vi "configure.vi"(8 "error in (no error)":errorcluster, 11 "DL090202FPGAClock in":refnum<class "ClockDL090202FPGA.lvclass">) -> (0 "error out":errorcluster, 3 "DL090202FPGAClock out":refnum<class "ClockDL090202FPGA.lvclass">)   [LabVIEW 2010, in "ClockDL090202FPGA.lvclass"]
uses:
  ClockDL090202FPGA.lvclass
  type_enum.ctl
  common/xcontrols/XComponentSpecification/XComponentSpecification/XComponentSpecification.xctl
  ClockDL090202FPGA.lvclass/ClockDL090202FPGA.ctl
  FPGAWrapper/GenericFPGAWrapper/GenericFPGAWrapper/GenericFPGAWrapper.lvclass
  common/classes/ErrorController/ErrorController/class_data.vi
  common/classes/GenericComponent/GenericComponent/GenericComponent.lvclass
  common/classes/ErrorController/ErrorController/ErrorController.lvclass
panel:
  in  "FPGAWrapper spec":T1(xcontrol)
  out "Configuration name":string
  in  "type":T2
  in  "cancel":bool
  in  "save":bool
  # "Configure ClockDL090202FPGA"
  # "FPGAWrapper"
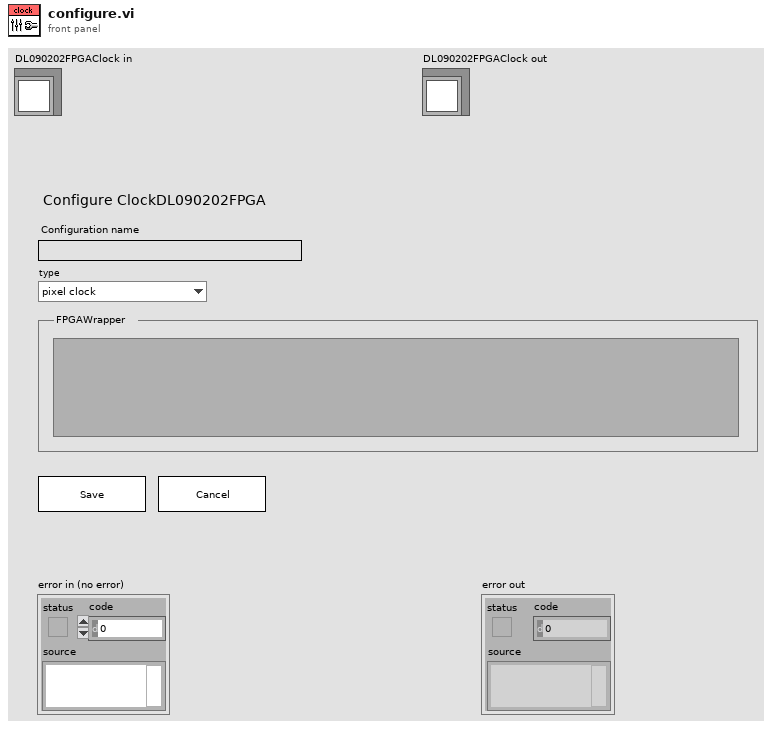
[diagram p1: front panel]
types:
  T1 = cluster{"class path":string, "configuration":string, "label":string, "settings name":string}
  T2 = typedef "ClockDL090202FPGA.lvclass/type_enum.ctl" = enum16{"pixel clock", "gate 1", "gate 2", "gate 3"}
  T3 = typedef "plugin_specification.ctl" = cluster{"class path":string, "configuration":string, "label":string, "settings name":string}
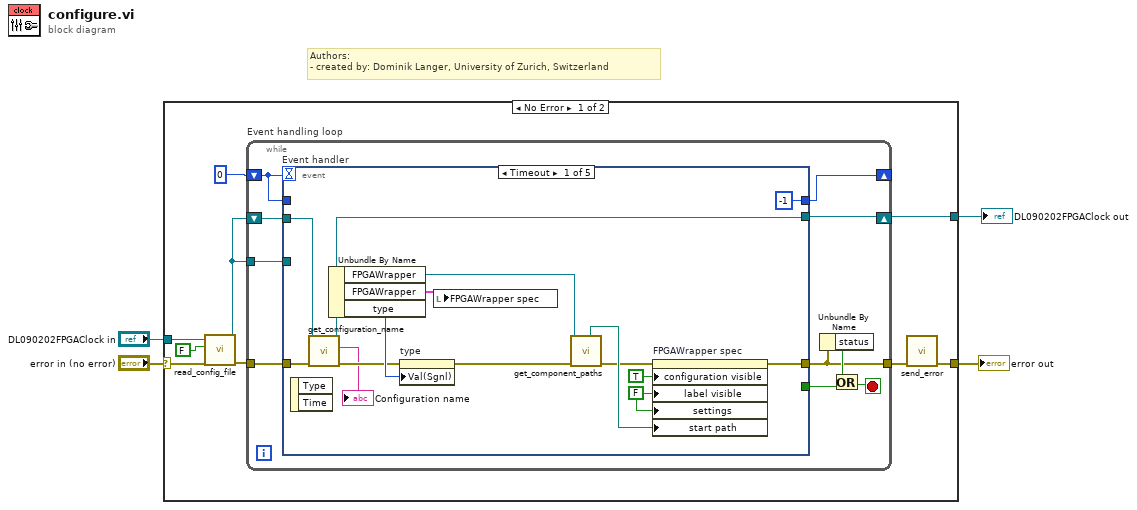
[diagram p0: block diagram]
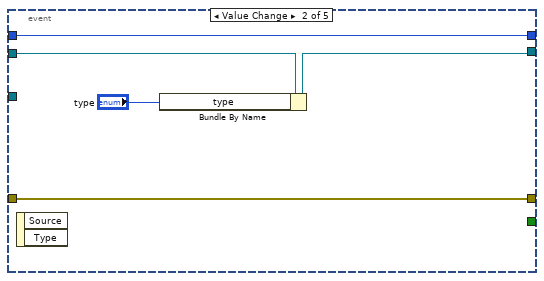
[diagram p2: hidden frame]
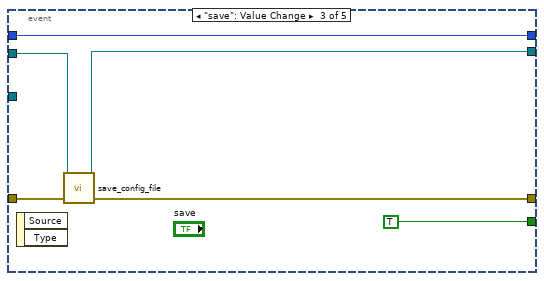
[diagram p3: hidden frame]
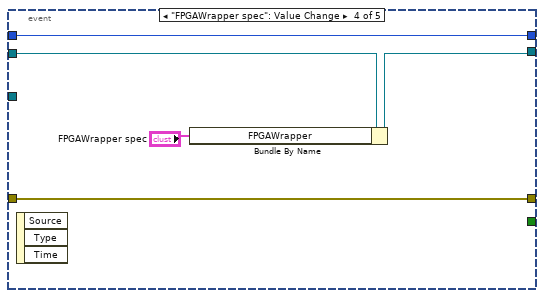
[diagram p4: hidden frame]
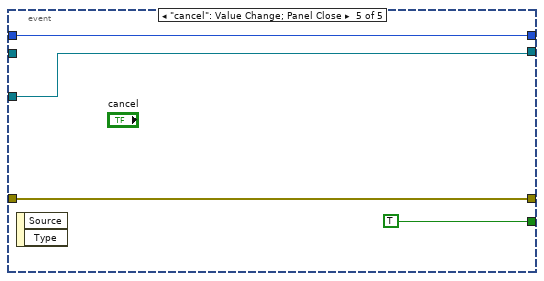
[diagram p5: hidden frame]
diagram:
  # "Authors: \n- created by: Dominik Langer, University of Zurich, Switzerland"
  n1 = case shown="No Error" "error in (no error)" {
    selector: "error in (no error)" -> [w11 w60]
    tunnel: [w7 w60] -> w3
    tunnel: [w12 w59] -> w1
    tunnel: "DL090202FPGAClock in" -> [w9 w59]
    frame No Error {
      n2 = call-dynamic "read_config_file.vi"("error in (no error)"=w11, "force load?"=FALSE, "GenericPlugin in"=w9) -> ("error out"=w10:errorcluster, "GenericPlugin out"=w5:refnum<class "ClockDL090202FPGA.lvclass">)  [unwired: 7 out]
      n3 = while "Event handling loop" {
        shift-right: [w21] -> _
        shift-left: 0 -> [w22]
        shift-right: [w19] -> w12
        shift-left: w5 -> [w20]
        tunnel: w10 -> [w23]
        tunnel: [w15] -> w6
        tunnel: w5 -> [w14]
        stop <- w17 stop-if-true
        n4 = event "Event handler" shown="[0] Timeout" {
          selector: _ -> [_ _ _ _ _]
          dyn-events: _ -> [_ _ _ _ _]
          timeout: w22 -> [_ _ _ _ _]
          tunnel: w23 -> [w36 w39 w48 w53 w57]
          tunnel: [-1 w43 w49 w54 w58] -> w21
          tunnel: w22 -> [_ w43 w49 w54 w58]
          tunnel: [w31 w39 w47 w53 w57] -> w15
          tunnel: [_ _ TRUE _ TRUE] -> w16
          tunnel: w20 -> [w34 w42 w44 w52 _]
          tunnel: [w25 w41 w46 w51 w55] -> w19
          tunnel: w14 -> [_ _ _ _ w55]
          event Timeout {
            w29 = FALSE ("label visible")
            n5 = event-data() -> ()  [unwired: 3 out]
            n6 = call "get_configuration_name.vi"("error in (no error)"=w36, "GenericPlugin.lvclass in"=w34) -> ("error out"=w35:errorcluster, "configuration name"=→"Configuration name":string, "GenericPlugin.lvclass out"=w25:refnum<class "ClockDL090202FPGA.lvclass">)  [unwired: 7 in]
            n7 = Unbundle By Name(w25) -> ("FPGAWrapper"=w24:refnum<class "GenericFPGAWrapper.lvclass">, "FPGAWrapper"=w32:T3, "type"=w37:T2)
            n8 = property on="type" class="Enum (strict)"(error in=w35, "Val(Sgnl)"=w37) -> (error out=w27:errorcluster)  [unwired: 1 in, 1 out]
            n9 = local write "FPGAWrapper spec"(w32) -> ()
            n10 = call-dynamic "get_component_paths.vi"("error in (no error)"=w27, "GenericComponent in"=w24) -> ("error out"=w26:errorcluster, "component type directory"=w28:path)  [unwired: 4 in, 4 out]
            n11 = property on="FPGAWrapper spec" class="XComponentSpecification (strict"(error in=w26, "configuration visible"=TRUE, "label visible"=w29, "settings"=w29, "start path"=w28) -> (error out=w31:errorcluster)  [unwired: 1 in, 1 out]
          }
          event Value Change {
            n12 = event-data() -> ()  [unwired: 3 out]
            n13 = Bundle By Name(cluster=w42, "type"="type") -> (w41:refnum<class "ClockDL090202FPGA.lvclass">)
          }
          event "save": Value Change {
            n14 = event-data() -> ()  [unwired: 3 out]
            n15 = call-dynamic "save_config_file.vi"("error in (no error)"=w48, "GenericPlugin in"=w44) -> ("error out"=w47:errorcluster, "GenericPlugin out"=w46:refnum<class "ClockDL090202FPGA.lvclass">)  [unwired: 2 in, 6 out]
          }
          event "FPGAWrapper spec": Value Change {
            n16 = event-data() -> ()  [unwired: 4 out]
            n17 = Bundle By Name(cluster=w52, "FPGAWrapper"="FPGAWrapper spec") -> (w51:refnum<class "ClockDL090202FPGA.lvclass">)
          }
          event "cancel": Value Change; Panel Close {
            n18 = event-data() -> ()  [unwired: 3 out]
          }
        }
        n19 = Unbundle By Name(w15) -> ("status"=w18:bool)
        n20 = Or(x=w18, y=w16) -> (x .or. y?=w17:bool)
      }
      n21 = call "send_error.vi"("error in (no error)"=w6) -> ("error out"=w7:errorcluster)  [unwired: 10 in]
    }
    frame Error {
    }
  }
  "error out" <- w3
  "DL090202FPGAClock out" <- w1
